vi "Stoppani_AvE.vi"(11 "file (use dialog)":path=path "/Users/crogers/Desktop/AVR read/Titian Strad All groups.AvC") -> (0 "run":cluster{"Sampling rate":u16, "Total time":dbl}, 1 "Complex FRF":cluster{"t0":dbl, "df":dbl, "Y":cdb[]}, 2 "TSingleArray":T1={"fComplex"=1, "fLength"=5166, "a[2]"=0.0, "fConditionCheck"=1, "Precision"=0.0, "MtxVecVersion"=420.0, "SizeOf(TSample)"=8.0, "Tag"=0.0, "MtxVecFileCode"=64019.0, "a[9]"=0.0, "a[10]"=0.0}, 3 "Header":T2 {"Average type" items=["RMS", "Mean", "Complex", "Geometric", "None"]; "dtAccel" items=["Accelerance", "Mobility", "Receptance", "Microphone", "Unknown"]})   [LabVIEW 2022 SP3]
uses:
  Stoppani_Ave_DataType.ctl
panel:
  out "caption":string
  out "String out":string
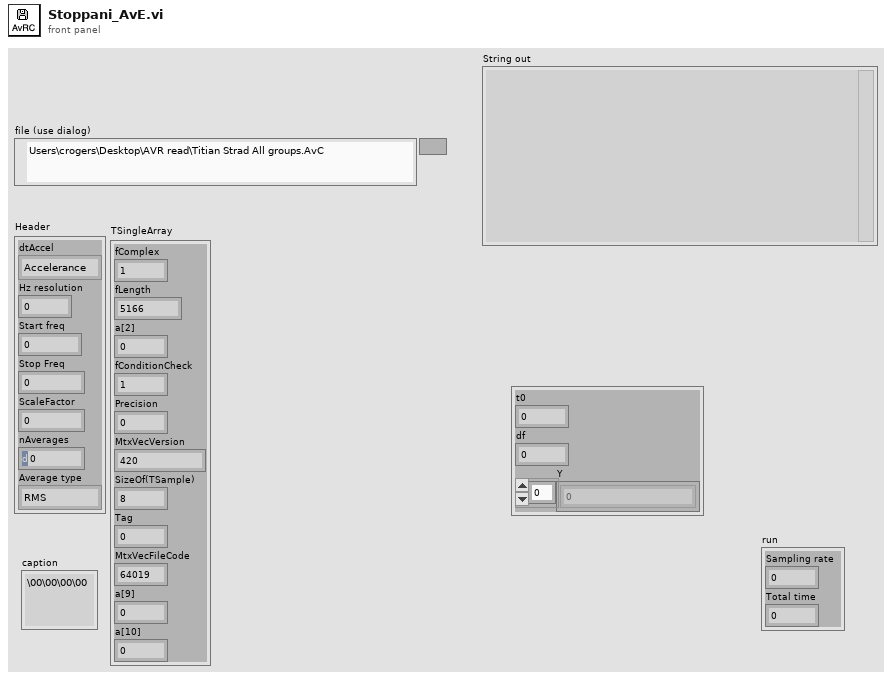
[diagram p1: front panel]
types:
  T1 = cluster{"fComplex":u32, "fLength":i32, "a[2]":dbl, "fConditionCheck":i16, "Precision":dbl, "MtxVecVersion":dbl, "SizeOf(TSample)":dbl, "Tag":dbl, "MtxVecFileCode":dbl, "a[9]":dbl, "a[10]":dbl}
  T2 = cluster{"dtAccel":u8, "Hz resolution":dbl, "Start freq":dbl, "Stop Freq":dbl, "ScaleFactor":dbl, "nAverages":u16, "Average type":u8}
  T3 = typedef "Stoppani_Ave_DataType.ctl" = enum16{"Char", "Byte", "Word", "Int", "Float (SGL)", "Float (DBL)", "Float (DBL Array)"}
  T4 = cluster{"[0]":dbl, "[1]":dbl, "[2]":dbl, "[3]":dbl, "[4]":dbl, "[5]":dbl, "[6]":dbl, "[7]":dbl, "[8]":dbl, "[9]":dbl, "[10]":dbl}
  T5 = cluster{"Start freq":dbl, "Hz resolution":dbl, cdb[]}
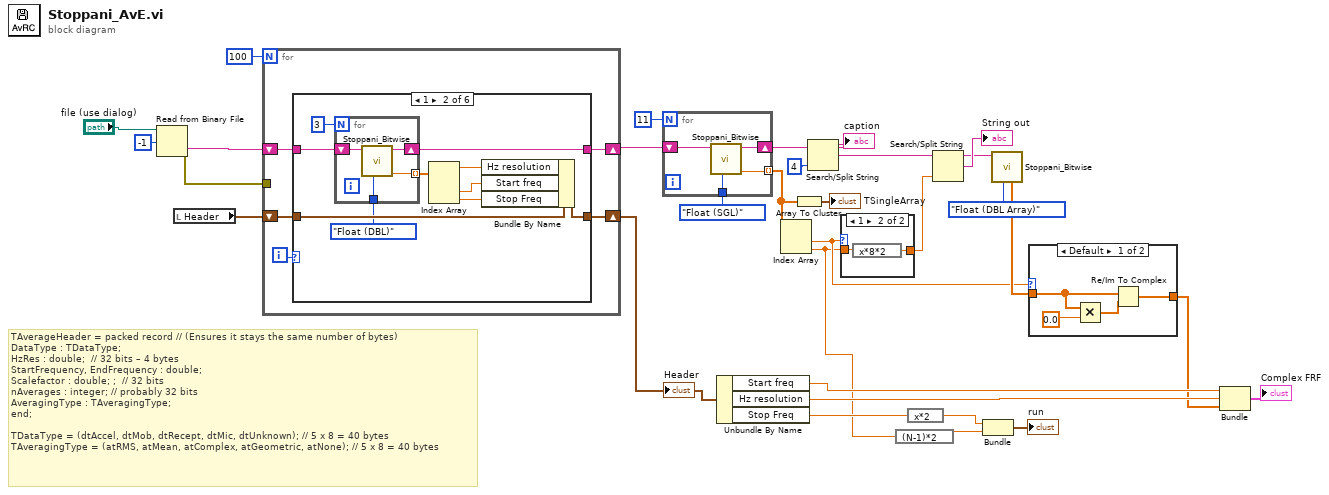
[diagram p0: block diagram]
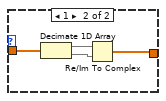
[diagram p2: hidden frame]
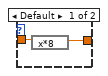
[diagram p3: hidden frame]
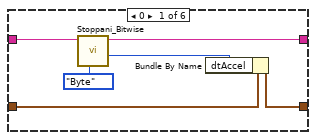
[diagram p4: hidden frame]
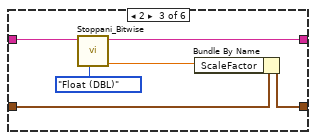
[diagram p5: hidden frame]
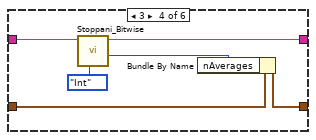
[diagram p6: hidden frame]
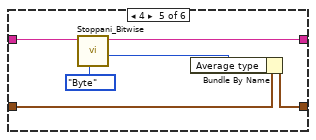
[diagram p7: hidden frame]
diagram:
  # "TAverageHeader = packed record // (Ensures it stays the same number of bytes)\nDataType : TDataType;\nHzRes : double;  // 32 bits – 4 bytes\nStartFrequency, EndFrequency : double;\nScalefactor : double; ;  // 32 bits\nnAverages : integer; // probably 32 bits\nAveragingType : TAveragingType;\nend;\n\nTDataType = (dtAccel, dtMob, dtRecept, dtMic, dtUnknown); // 5 x 8 = 40 bytes\nTAveragingType = (atRMS, atMean, atComplex, atGeometric, atNone); // 5 x 8 = 40 bytes"
  n1 = Read from Binary File(10:-1 ("count (1)"), 11:"file (use dialog)") -> (0:w9:errorcluster, 2:w27:string)  [unwired: 4 in, 2 out]
  n2 = local read "Header"() -> (w28:T2)
  n3 = for {
    N: 100 -> [_]
    shift-right: [w34] -> w24
    shift-left: w27 -> [w35]
    shift-right: [w33] -> w5
    shift-left: w28 -> [w32]
    tunnel: w9 -> [_]
    i -> [w36]
    n4 = case shown="1" w36 {
      tunnel: w35 -> [w42 w52 w62 w68 w74 w76]
      tunnel: [w41 w51 w61 w67 w73 w76] -> w34
      tunnel: [w39 w49 w59 w65 w71 w75] -> w33
      tunnel: w32 -> [w40 w50 w60 w66 w72 w75]
      frame 0 {
        n5 = call "Stoppani_Bitwise.vi"("Task"=Stoppani_Ave_DataType."Byte", "String In"=w42) -> ("Int"=w38:u32, "String Out"=w41:string)  [unwired: 5 in, 3 out]
        n6 = Bundle By Name(cluster=w40, "dtAccel"=w38) -> (w39:T2)
      }
      frame 1 {
        n7 = for {
          N: 3 -> [_]
          tunnel: [w54] -> w47 mode=indexing
          shift-right: [w55] -> w51
          shift-left: w52 -> [w56]
          tunnel: Stoppani_Ave_DataType."Float (DBL)" ("Task") -> [w53]
          n8 = call "Stoppani_Bitwise.vi"("Task"=w53, "String In"=w56) -> ("Float"=w54:dbl, "String Out"=w55:string)  [unwired: 5 in, 3 out]
        }
        n9 = Index Array(array=w47) -> (element #1=w46:dbl, element #2=w45:dbl, element #3=w44:dbl)  [unwired: 3 in]
        n10 = Bundle By Name(cluster=w50, "Hz resolution"=w46, "Start freq"=w45, "Stop Freq"=w44) -> (w49:T2)
      }
      frame 2 {
        n11 = call "Stoppani_Bitwise.vi"("Task"=Stoppani_Ave_DataType."Float (DBL)", "String In"=w62) -> ("Float"=w58:dbl, "String Out"=w61:string)  [unwired: 5 in, 3 out]
        n12 = Bundle By Name(cluster=w60, "ScaleFactor"=w58) -> (w59:T2)
      }
      frame 3 {
        n13 = call "Stoppani_Bitwise.vi"("Task"=Stoppani_Ave_DataType."Int", "String In"=w68) -> ("Int"=w64:u32, "String Out"=w67:string)  [unwired: 5 in, 3 out]
        n14 = Bundle By Name(cluster=w66, "nAverages"=w64) -> (w65:T2)
      }
      frame 4 {
        n15 = call "Stoppani_Bitwise.vi"("Task"=Stoppani_Ave_DataType."Byte", "String In"=w74) -> ("Int"=w70:u32, "String Out"=w73:string)  [unwired: 5 in, 3 out]
        n16 = Bundle By Name(cluster=w72, "Average type"=w70) -> (w71:T2)
      }
      frame Default {
      }
    }
  }
  "Header" <- w5
  n17 = for {
    N: 11 -> [_]
    shift-right: [w79] -> w23
    shift-left: w24 -> [w80]
    tunnel: [w78] -> w20 mode=indexing
    tunnel: Stoppani_Ave_DataType."Float (SGL)" ("Task") -> [w77]
    n18 = call "Stoppani_Bitwise.vi"("Task"=w77, "String In"=w80) -> ("Float"=w78:dbl, "String Out"=w79:string)  [unwired: 5 in, 3 out]
  }
  n19 = Unbundle By Name(w5) -> ("Start freq"=w22:dbl, "Hz resolution"=w21:dbl, "Stop Freq"=w4:dbl)
  n20 = Index Array(array=w20) -> (element #1=w10:dbl, element #2=w3:dbl)  [unwired: 2 in]
  n21 = Array To Cluster(array=w20) -> (cluster=→"TSingleArray":T4)
  n22 = Search/Split String(string=w23, offset (0)=4) -> (substring before match=→"caption":string, match + rest of string=w15:string)  [unwired: 1 in, 1 out]
  n23 = case shown="1" w10 {
    tunnel: w3 -> [w82 w84]
    tunnel: [w81 w83] -> w13
    frame Default {
      n24 = expression code="x*8"(w82) -> (w81:dbl)
    }
    frame 1 {
      n25 = expression code="x*8*2"(w84) -> (w83:dbl)
    }
  }
  n26 = expression code="(N-1)*2"(w3) -> (w2:dbl)
  n27 = expression code="x*2"(w4) -> (w6:dbl)
  n28 = Search/Split String(string=w15, offset (0)=w13) -> (substring before match=w12:string, match + rest of string=→"String out":string)  [unwired: 1 in, 1 out]
  n29 = Bundle("Stop Freq"=w6, "Float"=w2) -> (→"run":cluster{"Stop Freq":dbl, "Float":dbl})  [unwired: 1 in]
  n30 = call "Stoppani_Bitwise.vi"("Task"=Stoppani_Ave_DataType."Float (DBL Array)", "String In"=w12) -> ("Array"=w11:dbl[])  [unwired: 5 in, 4 out]
  n31 = case shown="Default" w10 {
    tunnel: w11 -> [w87 w90]
    tunnel: [w88 w89] -> w7
    frame Default {
      n32 = Multiply(x=w87, y=0.0 ("offset (0)")) -> (x*y=w86:dbl[])
      n33 = Re/Im To Complex(1:w86, 2:w87) -> (0:w88:cdb[])
    }
    frame 1 {
      n34 = Decimate 1D Array(w90) -> (w92:dbl[], w91:dbl[])
      n35 = Re/Im To Complex(1:w91, 2:w92) -> (0:w89:cdb[])
    }
  }
  n36 = Bundle("Start freq"=w22, "Hz resolution"=w21, w7) -> (→"Complex FRF":T5)  [unwired: 1 in]
